vi "inject_popup.vi"(10 "y_vals_IN":dbl[](array[numeric])=[1.0, 4.0, 9.0, 16.0, 25.0, 36.0, 49.0, 64.0, 81.0, 100.0]) -> (2 "y_vals":dbl[](array[numeric])=[1.0, 4.0, 9.0, 16.0, 12.0, 25.0, 36.0, 49.0, 64.0, 12.0, 81.0, 100.0], 3 "cancelled":bool)   [LabVIEW 2017, in "tools.lvlib"]
uses:
  tools.lvlib
  core/scan_inject.ctl
panel:
  in  "inject":T1={"inject_value"=99.0, "inject_every_n"=5, "inject_position"=enum."last"} {"inject_every_n" min=0; "inject_value" format="%#_6p"}
  in  "Cancel":bool
  in  "OK Button":bool
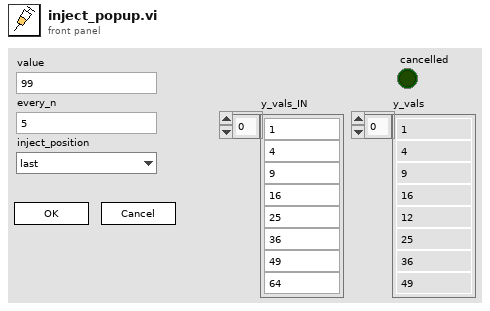
[diagram p1: front panel]
types:
  T1 = typedef "tools.lvlib/scan_inject.ctl" = cluster{"inject_value":dbl, "inject_every_n":i32, "inject_position":enum16{"first", "last"}}
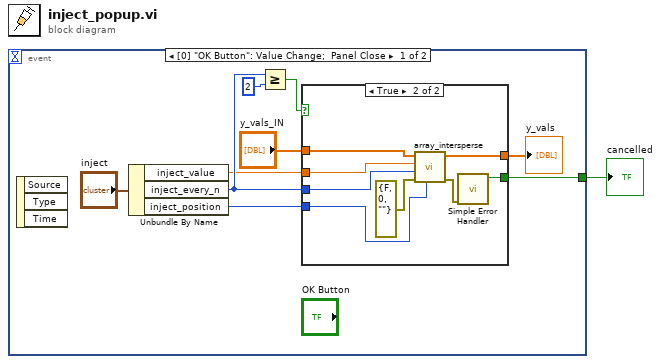
[diagram p0: block diagram]
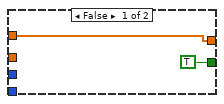
[diagram p2: hidden frame]
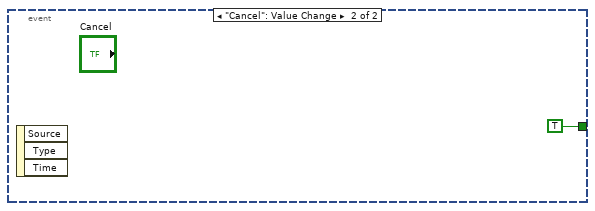
[diagram p3: hidden frame]
diagram:
  n1 = event shown="[0] \"OK Button\": Value Change;  Panel Close" {
    selector: _ -> [_ _]
    dyn-events: _ -> [_ _]
    timeout: _ -> [_ _]
    tunnel: [w2 TRUE ("Cancel")] -> w1
    event "OK Button": Value Change; Panel Close {
      n2 = event-data() -> ()  [unwired: 1 in, 3 out]
      n3 = Unbundle By Name("inject") -> ("inject_value"=w6:dbl, "inject_every_n"=w7:i32, "inject_position"=w8:enum16{"first", "last"})
      n4 = Greater Or Equal?(x=w7, y=2) -> (x >= y?=w9:bool)
      n5 = case shown="True" w9 {
        tunnel: "y_vals_IN" -> [w12 w20]
        tunnel: [w12 w19] -> w3
        tunnel: w6 -> [_ w18]
        tunnel: w7 -> [_ w17]
        tunnel: w8 -> [_ w14]
        tunnel: [TRUE ("error?") w13] -> w2
        frame False {
        }
        frame True {
          n6 = call "array_intersperse.vi"("position"=w14, "error in"=errorcluster {"status"=FALSE, "code"=0, "source"=""}, "every"=w17, "inject value"=w18, "input_values"=w20) -> ("error out"=w16:errorcluster, "result"=w19:dbl[])  [unwired: 3 in, 2 out]
          n7 = call <vilib>:"Simple Error Handler.vi"("error in (no error)"=w16) -> ("error?"=w13:bool)  [unwired: 4 in, 4 out]
        }
      }
      "y_vals" <- w3
    }
    event "Cancel": Value Change {
      n8 = event-data() -> ()  [unwired: 1 in, 3 out]
    }
  }
  "cancelled" <- w1
